vi "Read viancfg Items to Analyze.vi"(8 "Error in":errorcluster caption="Error in (no error)", 11 "viancfg Path":path) -> (0 "Error out":errorcluster, 2 "Included Paths":path[](array[path]), 3 "Removed Paths":path[](array[path]))   [LabVIEW 2023]
uses:
  <vilib>/xml/Load XML File.vi
  <vilib>/xml/Close Reference(Node).vi
  <vilib>/xml/NI_XML.lvlib
  <resource>/objmgr/DOMUserDefRef.rc
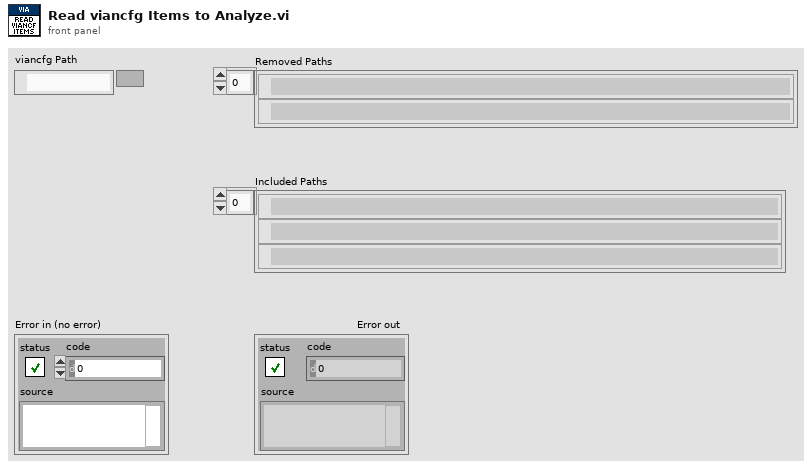
[diagram p1: front panel]
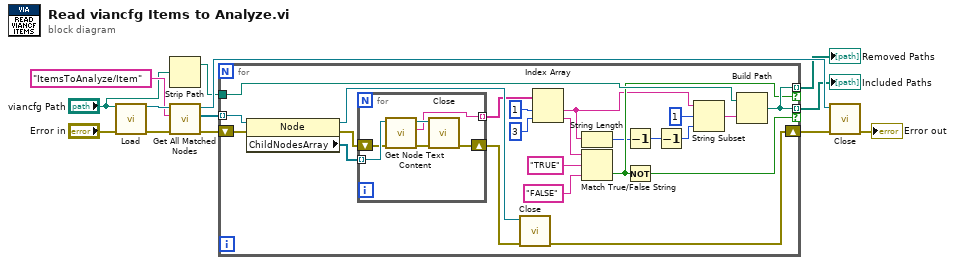
[diagram p0: block diagram]
diagram:
  n1 = call-poly <vilib>:"Load.vi"("path to XML document"="viancfg Path", "error in (no error)"="Error in") -> ("DOM document out"=w13:refnum<k20>, "error out"=w12:errorcluster)  [unwired: 11 in, 1 out]
  n2 = Strip Path(path="viancfg Path") -> (stripped path=w6:path)  [unwired: 1 out]
  n3 = call <vilib>:"Get All Matched Nodes.vi"("error in (no error)"=w12, "XPath expression"="ItemsToAnalyze/Item", "node in"=w13) -> ("error out"=w10:errorcluster, "node result array"=w9:refnum<k20>[], "node out"=w8:refnum<k20>)  [unwired: 6 in]
  n4 = for {
    tunnel: w9 -> [w36] mode=indexing
    shift-right: [w14] -> w7
    shift-left: w10 -> [w34]
    tunnel: w6 -> [w25]
    tunnel: [w24] -> w5 mode=indexing if=w23
    tunnel: [w24] -> w4 mode=indexing if=w22
    n5 = property class="Node"(reference=w36, error in=w34) -> (reference out=w35:refnum<k20>, error out=w32:errorcluster, "ChildNodesArray"=w33:refnum<k20>[])
    n6 = for {
      tunnel: w33 -> [w41] mode=indexing
      tunnel: [w37] -> w31 mode=indexing
      shift-right: [w42] -> w15
      shift-left: w32 -> [w40]
      n7 = call <vilib>:"Get Node Text Content.vi"("error in (no error)"=w40, "node in"=w41) -> ("error out"=w38:errorcluster, "node text"=w37:string, "node out"=w39:refnum<k20>)  [unwired: 7 in]
      n8 = call-poly <vilib>:"Close.vi"("error in (no error)"=w38, "node"=w39) -> ("error out"=w42:errorcluster)  [unwired: 7 out]
    }
    n9 = call-poly <vilib>:"Close.vi"("error in (no error)"=w15, "node"=w35) -> ("error out"=w14:errorcluster)  [unwired: 7 out]
    n10 = Index Array(array=w31, index #1=1 ("index"), index #2=3 ("index")) -> (element #1=w18:string, element #2=w28:string)
    n11 = String Length(string=w18) -> (length=w20:i32)
    n12 = Match True/False String(2:"FALSE" ("false string"), 3:"TRUE" ("true string"), 4:w28) -> (0:w23:bool)  [unwired: 1 out]
    n13 = Decrement(x=w20) -> (x-1=w19:i32)
    n14 = Not(x=w23) -> (.not. x?=w22:bool)
    n15 = Decrement(x=w19) -> (x-1=w16:i32)
    n16 = String Subset(string=w18, offset (0)=1, length (rest)=w16) -> (substring=w17:string)
    n17 = Build Path(base path=w25, name or relative path=w17) -> (appended path=w24:path)
  }
  "Removed Paths" <- w5
  "Included Paths" <- w4
  n18 = call-poly <vilib>:"Close.vi"("error in (no error)"=w7, "node"=w8) -> ("error out"=→"Error out":errorcluster)  [unwired: 7 out]
